vi "IB_RW_Project_Shortcut.vi"(7 "action":T3, 8 "error in (no error)":errorcluster, 9 "index in":string, 10 "dataSource in":T2, 11 "buildObject":T1) -> (0 "error out":errorcluster, 1 "index out":string, 2 "dataSource out":T2, 3 "buildObject out":T1)   [LabVIEW 2020]
doc: "Reads and writes the data to the object property bag."
uses:
  <resource>/Framework/Providers/API/ItemRef.ctl
  <vilib>/AppBuilder/IB_RW_Project/IB_RW_Project_PropBag_Action.ctl
  <vilib>/AppBuilder/IB_RW_Project/IB_RW_Project_Shortcut_Data.ctl
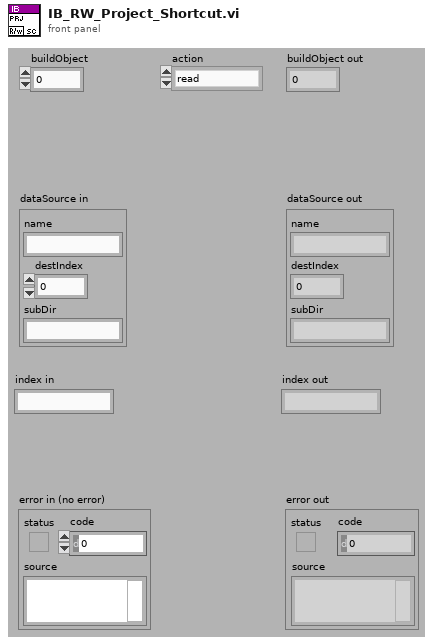
[diagram p1: front panel]
types:
  T1 = typedef "ItemRef.ctl" = u64
  T2 = typedef "IB_RW_Project_Shortcut_Data.ctl" = cluster{"name":string, "destIndex":i32, "subDir":string}
  T3 = typedef "IB_RW_Project_PropBag_Action.ctl" = enum16{"read", "write", "clear", "readPrevious", "writePrevious", "clearPrevious"}
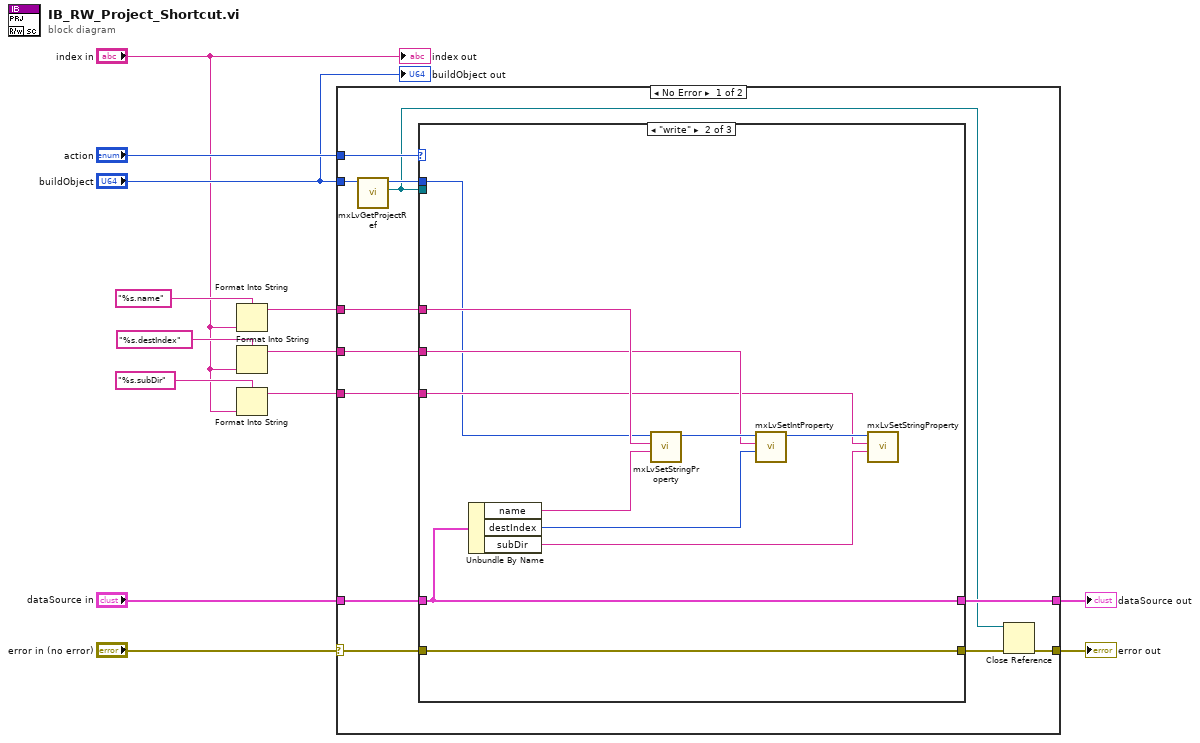
[diagram p0: block diagram]
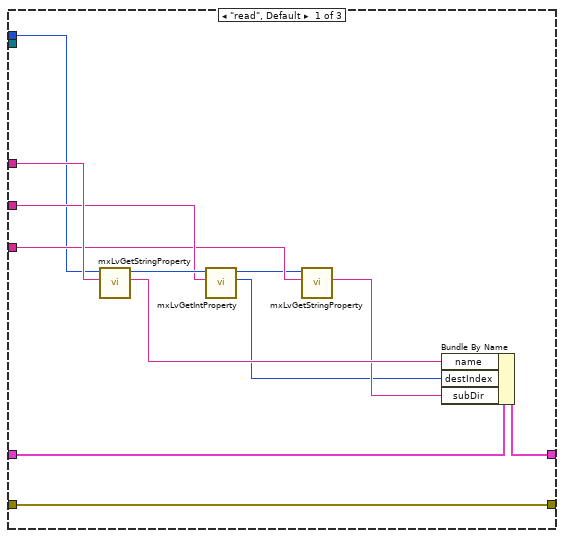
[diagram p2: hidden frame]
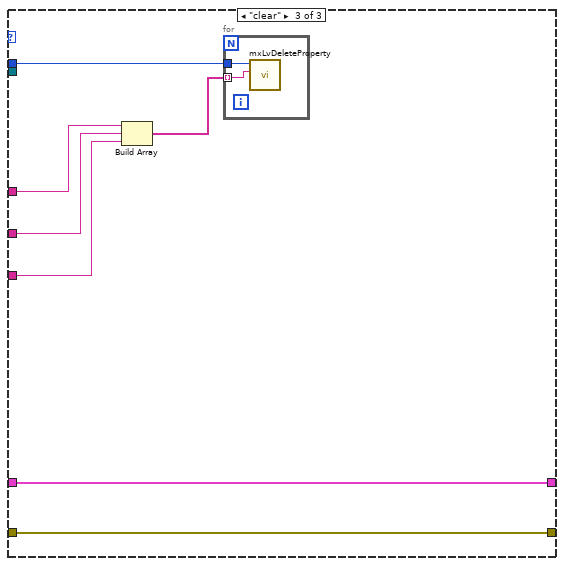
[diagram p3: hidden frame]
diagram:
  n1 = Format Into String(format string="%s.name", "index in") -> (resulting string=w4:string)  [unwired: 2 in, 1 out]
  n2 = Format Into String(format string="%s.destIndex", "index in") -> (resulting string=w7:string)  [unwired: 2 in, 1 out]
  n3 = Format Into String(format string="%s.subDir", "index in") -> (resulting string=w5:string)  [unwired: 2 in, 1 out]
  n4 = case shown="No Error" "error in (no error)" {
    selector: "error in (no error)" -> [w17 w58]
    tunnel: "action" -> [w25 _]
    tunnel: "dataSource in" -> [w24 w59]
    tunnel: [w23 w59] -> w11
    tunnel: "buildObject" -> [w19 _]
    tunnel: w7 -> [w22 _]
    tunnel: w5 -> [w21 _]
    tunnel: w4 -> [w20 _]
    tunnel: [w15 w58] -> w2
    frame No Error {
      n5 = call <resource>:"mxLvGetProjectRef.vi"("Item"=w19) -> ("Project Refnum"=w14:refnum<vi>, "Item"=w18:T1)  [unwired: 1 in, 8 out]
      n6 = case shown="\"write\"" w25 {
        tunnel: w18 -> [w27 w39 w49]
        tunnel: w24 -> [w37 w48 w55]
        tunnel: [w36 w48 w55] -> w23
        tunnel: w22 -> [w32 w43 w53]
        tunnel: w21 -> [w31 w40 w52]
        tunnel: w20 -> [w34 w45 w51]
        tunnel: [w28 w47 w50] -> w16
        tunnel: w17 -> [w28 w47 w50]
        tunnel: w14 -> [_ _ _]
        frame "read", Default {
          n7 = call <resource>:"mxLvGetStringProperty.vi"("Tag"=w34, "Item"=w27) -> ("Value"=w35:string, "Item"=w33:T1)  [unwired: 1 in, 7 out]
          n8 = call <resource>:"mxLvGetIntProperty.vi"("Tag"=w32, "Item"=w33) -> ("Value"=w26:i32, "Item"=w30:T1)  [unwired: 1 in, 7 out]
          n9 = call <resource>:"mxLvGetStringProperty.vi"("Tag"=w31, "Item"=w30) -> ("Value"=w29:string)  [unwired: 1 in, 8 out]
          n10 = Bundle By Name(cluster=w37, "name"=w35, "destIndex"=w26, "subDir"=w29) -> (w36:T2)
        }
        frame "write" {
          n11 = Unbundle By Name(w48) -> ("name"=w46:string, "destIndex"=w38:i32, "subDir"=w41:string)
          n12 = call <resource>:"mxLvSetStringProperty.vi"("Value (\"\")"=w46, "Tag"=w45, "Item"=w39) -> ("Item"=w44:T1)  [unwired: 2 in, 6 out]
          n13 = call <resource>:"mxLvSetIntProperty.vi"("Value (0)"=w38, "Tag"=w43, "Item"=w44) -> ("Item"=w42:T1)  [unwired: 3 in, 5 out]
          n14 = call <resource>:"mxLvSetStringProperty.vi"("Value (\"\")"=w41, "Tag"=w40, "Item"=w42) -> ()  [unwired: 2 in, 7 out]
        }
        frame "clear" {
          n15 = Build Array(w51, w53, w52) -> (w54:string[])
          n16 = for {
            tunnel: w54 -> [w57] mode=indexing
            tunnel: w49 -> [w56]
            n17 = call <resource>:"mxLvDeleteProperty.vi"("Tag"=w57, "Item"=w56) -> ()  [unwired: 1 in, 9 out]
          }
        }
      }
      n18 = Close Reference(reference=w14, error in (no error)=w16) -> (error out=w15:errorcluster)
    }
    frame Error {
    }
  }
  "error out" <- w2
  "dataSource out" <- w11
  "buildObject out" <- "buildObject"
  "index out" <- "index in"
